vi "Stop Core.vi"(10 "final error code":i32, 11 "System Actor in":refnum<class "System Actor.lvclass">) -> (3 "System Actor out":refnum<class "System Actor.lvclass">)   [LabVIEW 2013, in "Robot Actors.lvlib" / "System Actor.lvlib" / "System Actor.lvclass"]
doc: "(<B>Filename</B>: Actor Framework.lvlib:Actor.lvclass:Stop Core.vi)\n\nDefines what the actor does before it stops. Use the <B>final error code</B> input to determine whether the actor shut down in response to an error.\n\nBy default, this method does nothing. A descendant class may override it to define behavior, such as shutting down any processes the actor initiated in its override of the Actor Core method."
uses:
  System Actor.lvclass
  System Actor.lvclass/System Actor.ctl
  State Actor/State Actor.lvclass
  <vilib>/ActorFramework/Stop Msg/Stop Msg.lvclass/Stop Msg.ctl
  <vilib>/ActorFramework/Message Enqueuer/Message Enqueuer.lvclass/Message Enqueuer.ctl
  <vilib>/ActorFramework/Stop Msg/Send Emergency Stop.vi
  <vilib>/ActorFramework/Stop Msg/Send Normal Stop.vi
  <vilib>/ActorFramework/Message Enqueuer/Enqueue Critical.vi
  <vilib>/ActorFramework/Message Enqueuer/Enqueue.vi
  <vilib>/ActorFramework/Message Priority Queue/Priority Enqueue.vi
  <vilib>/ActorFramework/Stop Msg/Stop Msg.lvclass
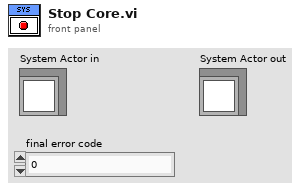
[diagram p1: front panel]
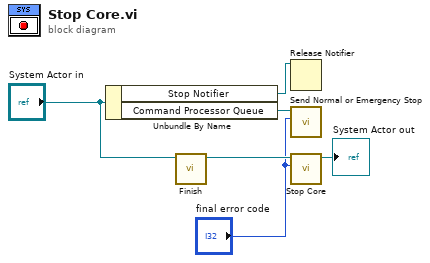
[diagram p0: block diagram]
diagram:
  n1 = Unbundle By Name("System Actor in") -> ("Stop Notifier"=w3:refnum<notifier>, "Command Processor Queue"=w2:refnum<class "Message Enqueuer.lvclass">)
  n2 = call-dynamic "Finish.vi"("System Actor in"="System Actor in") -> ("System Actor out"=w5:refnum<class "System Actor.lvclass">)  [unwired: 9 in, 1 out]
  n3 = Release Notifier(notifier=w3) -> ()  [unwired: 2 in, 3 out]
  n4 = call <vilib>:"Send Normal or Emergency Stop.vi"("final error code"="final error code", "Message Enqueuer"=w2) -> ()  [unwired: 9 in, 1 out]
  n5 = call-parent "Stop Core.vi"("final error code"="final error code", "Actor in"=w5) -> ("Actor out"=→"System Actor out":refnum<class "System Actor.lvclass">)  [unwired: 9 in]
